vi "Data.vi"(11 "Last Ack Msg in":refnum<class "Last Ack Msg.lvclass">) -> (2 "Queue Actor":refnum<class "Queue Actor.lvclass">)   [LabVIEW 2021, in "Last Ack.lvlib" / "Last Ack Msg.lvclass"]
uses:
  Last Ack Msg.lvclass
  Queue Actor/Queue Actor.lvclass
  Last Ack Msg.lvclass/Last Ack Msg.ctl
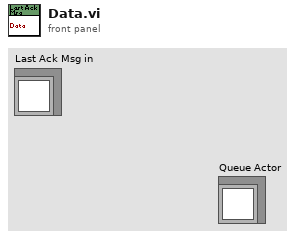
[diagram p1: front panel]
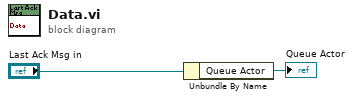
[diagram p0: block diagram]
diagram:
  n1 = Unbundle By Name("Last Ack Msg in") -> ("Queue Actor"=→"Queue Actor":refnum<class "Queue Actor.lvclass">)
